vi "MGCC_StaEst_WeightMatrix.vi"(1 "MeaIdx":cluster{"PN":dbl[], "QN":dbl[], "VN":dbl[]}, 2 "SensorError":cluster{"PN":dbl, "QN":dbl, "VN":dbl}) -> (0 "R":dbl[][](array[numeric]))   [LabVIEW 2016]
uses:
  <vilib>/imath/engines/lvmath2/RunTimeEngine/RunTimeType/NIMS_RunTimeType_From StrictType (excl LVString).vi
  <instcachedir>/0/NIMS_RunTimeType_From StrictType (excl LVString)_BBF44FB49F834B71AF7A14CCEDF8BECD.lvgen/NIMS_RunTimeType_From StrictType (excl LVString)_BBF44FB49F834B71AF7A14CCEDF8BECD_031.vi
  <vilib>/imath/engines/lvmath2/RunTimeEngine/Struct/NIMS_StructSetField.vi
  <vilib>/imath/engines/lvmath2/RunTimeEngine/Struct/NIMS_StructGetField.vi
  <vilib>/imath/engines/lvmath2/RunTimeEngine/RunTimeType/NIMS_RunTimeType_To Numeric.vi
  <instcachedir>/0/NIMS_RunTimeType_To Numeric_19D51BCABB82435A94073491761E42EE.lvgen/NIMS_RunTimeType_To Numeric_19D51BCABB82435A94073491761E42EE_008.vi
  <instcachedir>/0/NIMS_RunTimeType_From StrictType (excl LVString)_BBF44FB49F834B71AF7A14CCEDF8BECD.lvgen/NIMS_RunTimeType_From StrictType (excl LVString)_BBF44FB49F834B71AF7A14CCEDF8BECD_010.vi
  <instcachedir>/0/NIMS_RunTimeType_To Numeric_19D51BCABB82435A94073491761E42EE.lvgen/NIMS_RunTimeType_To Numeric_19D51BCABB82435A94073491761E42EE_004.vi
  <vilib>/imath/engines/lvmath2/RunTimeEngine/BuiltInFunctions/size/NIMS_I32Row=size(GRow).vi
  <instcachedir>/0/NIMS_I32Row=size(GRow)_E5C05C6B13124B29B774CC4F993D3C59.lvgen/NIMS_I32Row=size(GRow)_E5C05C6B13124B29B774CC4F993D3C59_000.vi
  <vilib>/imath/engines/lvmath2/RunTimeEngine/BuiltInFunctions/ones/NIMS_M=ones(I32V).vi
  <vilib>/imathl/engines/lvmath/Functions/Error Handling/Create Error.vi
  <vilib>/imath/engines/lvmath2/RunTimeEngine/RowToken/NIMS_RowToken_M_M.vi
  <instcachedir>/0/NIMS_RowToken_M_M_968CDE3545E74ACDAEA4B48DE01EEECA.lvgen/NIMS_RowToken_M_M_968CDE3545E74ACDAEA4B48DE01EEECA_004.vi
  <vilib>/imath/engines/lvmath2/RunTimeEngine/BuiltInFunctions/diag/NIMS_diag.vi
  <instcachedir>/0/NIMS_diag_BAFF033CE85645D0951408836EA255EA.lvgen/NIMS_diag_BAFF033CE85645D0951408836EA255EA_003.vi
  <vilib>/imath/engines/lvmath2/RunTimeEngine/ErrorHandling/NIMS_Create Error From Enums.vi
  <vilib>/imath/engines/lvmath2/RunTimeEngine/NodeEndStatement/NIMS_NodeEndStatement_Output.vi
  <instcachedir>/0/NIMS_NodeEndStatement_Output_53EC0D466D134D7ABD903AC30B43404B.lvgen/NIMS_NodeEndStatement_Output_53EC0D466D134D7ABD903AC30B43404B_002.vi
  <instcachedir>/0/NIMS_NodeEndStatement_Output_53EC0D466D134D7ABD903AC30B43404B.lvgen/NIMS_NodeEndStatement_Output_53EC0D466D134D7ABD903AC30B43404B_024.vi
  <instcachedir>/0/NIMS_NodeEndStatement_Output_53EC0D466D134D7ABD903AC30B43404B.lvgen/NIMS_NodeEndStatement_Output_53EC0D466D134D7ABD903AC30B43404B_025.vi
  <vilib>/imath/engines/lvmath2/RunTimeEngine/ErrorHandling/NIMS_Finalize Error.vi
panel:
  out "WVN":dbl[][](array[numeric])
  out "WQN":dbl[][](array[numeric])
  out "WPN":dbl[][](array[numeric])
  out "error out":errorcluster
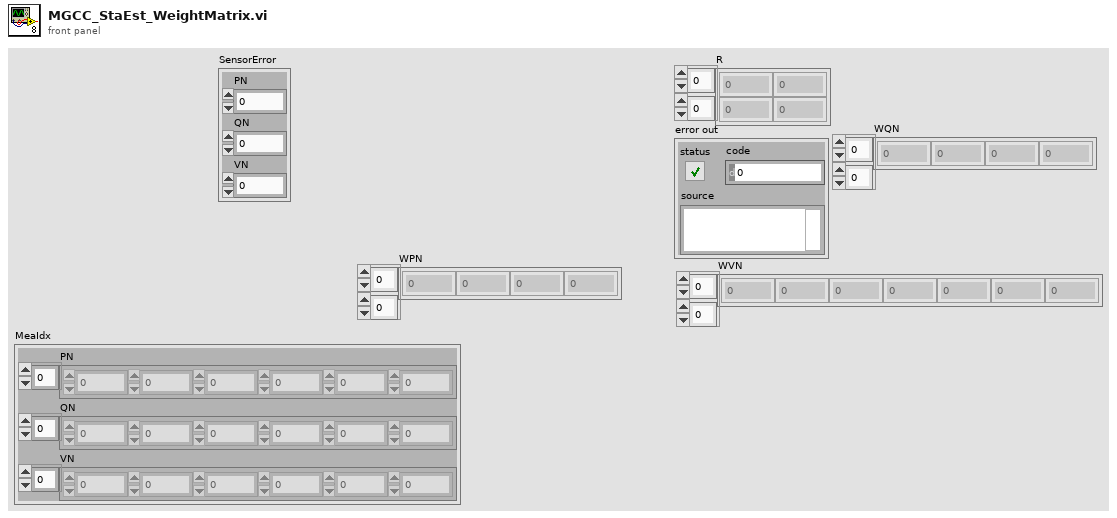
[diagram p1: front panel]
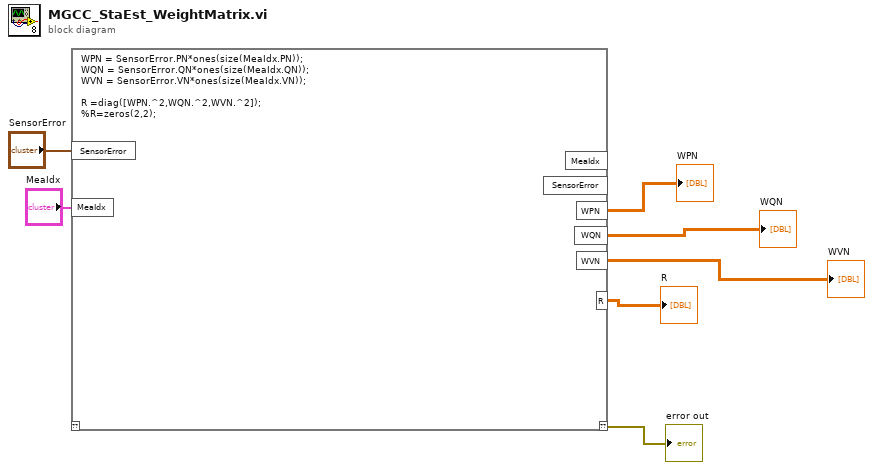
[diagram p0: block diagram]
diagram:
  n1 = mathscript code="WPN = SensorError.PN*ones(size(MeaIdx.PN));\nWQN = SensorError.QN*ones(size(MeaIdx.QN));\nWVN = SensorError.VN*ones(size(MeaIdx.VN));\n\nR =diag([WPN.^2,WQN.^2,WVN.^2]);\n%R=zeros(2,2);"("MeaIdx"="MeaIdx", "SensorError"="SensorError") -> ("??"=→"error out":errorcluster, "R"=→"R":dbl[][], "WPN"=→"WPN":dbl[][], "WQN"=→"WQN":dbl[][], "WVN"=→"WVN":dbl[][])  [unwired: 1 in, 2 out]
